vi "_sub_balance.vi"(11 "클러스터":T1) -> (2 "Balance xy wfs":cluster{"X":dbl, "Y":dbl}[](graph), 3 "Balance":cluster{"X":dbl, "Y":dbl}[](graph))   [LabVIEW 2013]
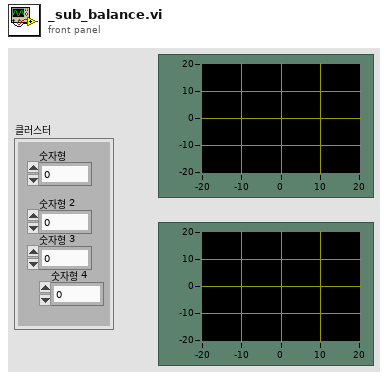
[diagram p1: front panel]
types:
  T1 = cluster{"숫자형":dbl, "숫자형 2":dbl, "숫자형 3":dbl, "숫자형 4":dbl}
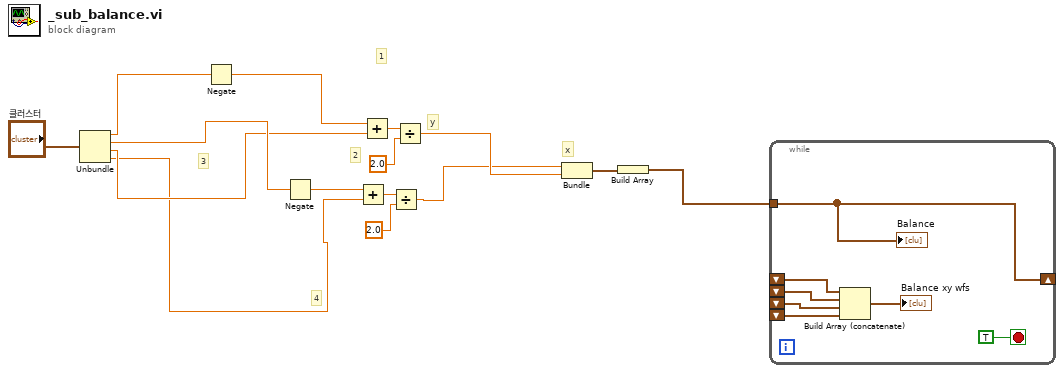
[diagram p0: block diagram]
diagram:
  # "y"
  # "x"
  # "4"
  # "3"
  # "2"
  # "1"
  n1 = Unbundle("클러스터") -> ("숫자형"=w4:dbl, "숫자형 2"=w3:dbl, "숫자형 3"=w2:dbl, "숫자형 4"=w1:dbl)
  n2 = Negate(x=w4) -> (-x=w14:dbl)
  n3 = Negate(x=w3) -> (-x=w15:dbl)
  n4 = Add(x=w15, y=w1) -> (x+y=w10:dbl)
  n5 = Add(x=w14, y=w2) -> (x+y=w12:dbl)
  n6 = Divide(x=w10, y=2.0) -> (x/y=w7:dbl)
  n7 = Divide(x=w12, y=2.0) -> (x/y=w8:dbl)
  n8 = Bundle(w7, w8) -> (w9:cluster{dbl, dbl})  [unwired: 1 in]
  n9 = Build Array(w9) -> (w6:cluster{dbl, dbl}[])
  n10 = while {
    shift-right: [w21] -> _
    shift-left: _ -> [w17]
    tunnel: w6 -> [w21]
    shift-left: _ -> [w18]
    shift-left: _ -> [w19]
    shift-left: _ -> [w20]
    stop <- TRUE stop-if-true
    n11 = Build Array (concatenate)(w17, w18, w19, w20) -> (→"Balance xy wfs":cluster{dbl, dbl}[])
    "Balance" <- w21
  }
